vi "DEMO.vi"() -> ()   [LabVIEW 2011]
panel:
  in  "主轴停止":bool
  in  "主轴启动":bool
  in  "关灯":bool
  in  "开灯":bool
  in  "关闭冷却":bool
  in  "打开冷却":bool
  in  "停止":bool
  out "Output":string
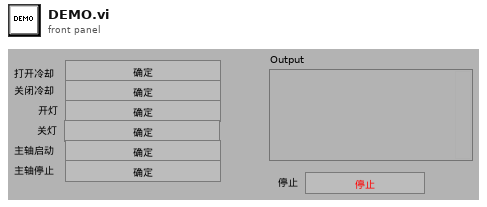
[diagram p1: front panel]
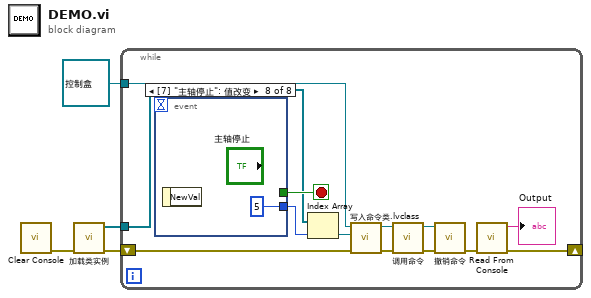
[diagram p0: block diagram]
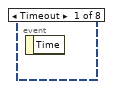
[diagram p2: hidden frame]
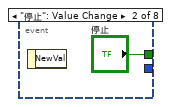
[diagram p3: hidden frame]
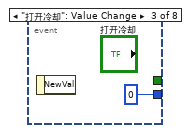
[diagram p4: hidden frame]
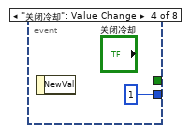
[diagram p5: hidden frame]
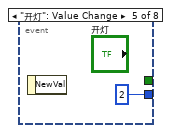
[diagram p6: hidden frame]
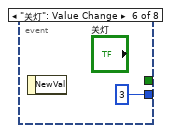
[diagram p7: hidden frame]
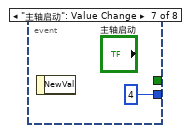
[diagram p8: hidden frame]
diagram:
  n1 = call "Clear Console.vi"() -> ("error out"=w3:errorcluster)  [unwired: 11 in]
  n2 = call "加载类实例.vi"("error in (no error)"=w3) -> ("error out"=w2:errorcluster, "数组"=w1:refnum<class "命令类.lvclass">[])  [unwired: 9 in]
  n3 = while {
    tunnel: refnum<class "控制盒.lvclass"> refnum ("控制盒.lvclass") -> [w13]
    shift-right: [w7] -> _
    shift-left: w2 -> [w8]
    tunnel: w1 -> [w6]
    stop <- w17 stop-if-true
    n4 = event shown="[7] \"主轴停止\": 值改变" {
      selector: _ -> [_ _ _ _ _ _ _ _]
      dyn-events: _ -> [_ _ _ _ _ _ _ _]
      timeout: _ -> [_ _ _ _ _ _ _ _]
      tunnel: [_ "停止" _ _ _ _ _ _] -> w17
      tunnel: [_ _ 0 ("索引") 1 ("索引") 2 ("索引") 3 ("索引") 4 ("索引") 5 ("索引")] -> w12
      event Timeout {
        n5 = event-data() -> ()  [unwired: 1 in, 1 out]
      }
      event "停止": Value Change {
        n6 = event-data() -> ()  [unwired: 1 in, 1 out]
      }
      event "打开冷却": Value Change {
        n7 = event-data() -> ()  [unwired: 1 in, 1 out]
      }
      event "关闭冷却": Value Change {
        n8 = event-data() -> ()  [unwired: 1 in, 1 out]
      }
      event "开灯": Value Change {
        n9 = event-data() -> ()  [unwired: 1 in, 1 out]
      }
      event "关灯": Value Change {
        n10 = event-data() -> ()  [unwired: 1 in, 1 out]
      }
      event "主轴启动": Value Change {
        n11 = event-data() -> ()  [unwired: 1 in, 1 out]
      }
      event "主轴停止": Value Change {
        n12 = event-data() -> ()  [unwired: 1 in, 1 out]
      }
    }
    n13 = Index Array(array=w6, index=w12) -> (element=w5:refnum<class "命令类.lvclass">)
    n14 = call "写入命令类.lvclass.vi"("error in (no error)"=w8, "命令类.lvclass"=w5, "控制盒输入"=w13) -> ("error out"=w16:errorcluster, "控制盒输出"=w15:refnum<class "控制盒.lvclass">)  [unwired: 7 in]
    n15 = call "调用命令.vi"("error in (no error)"=w16, "控制盒 输入"=w15) -> ("error out"=w10:errorcluster, "控制盒 输出"=w11:refnum<class "控制盒.lvclass">)  [unwired: 8 in]
    n16 = call "撤销命令.vi"("error in (no error)"=w10, "控制盒 输入"=w11) -> ("error out"=w9:errorcluster)  [unwired: 8 in, 1 out]
    n17 = call "Read From Console.vi"("error in (no error)"=w9) -> ("error out"=w7:errorcluster, "Output"=→"Output":string)  [unwired: 9 in]
  }
